vi "Test Set Base Path.vi"() -> ()   [LabVIEW 2021, in "Path Utilities.lvlib"]
doc: "Unit Test for \"Get In AppData Local.vi\"."
uses:
  Path Utilities.lvlib
panel:
  out "Pass":bool[](array[boolean])
  out "Result - System Paths with Base":path[](array[path])
  out "Expected - System Paths with Base":path[](array[path])
  in  "User Name":string="Thomas"
  out "error out":errorcluster
  in  "Base Path":path=path "Company/Application"
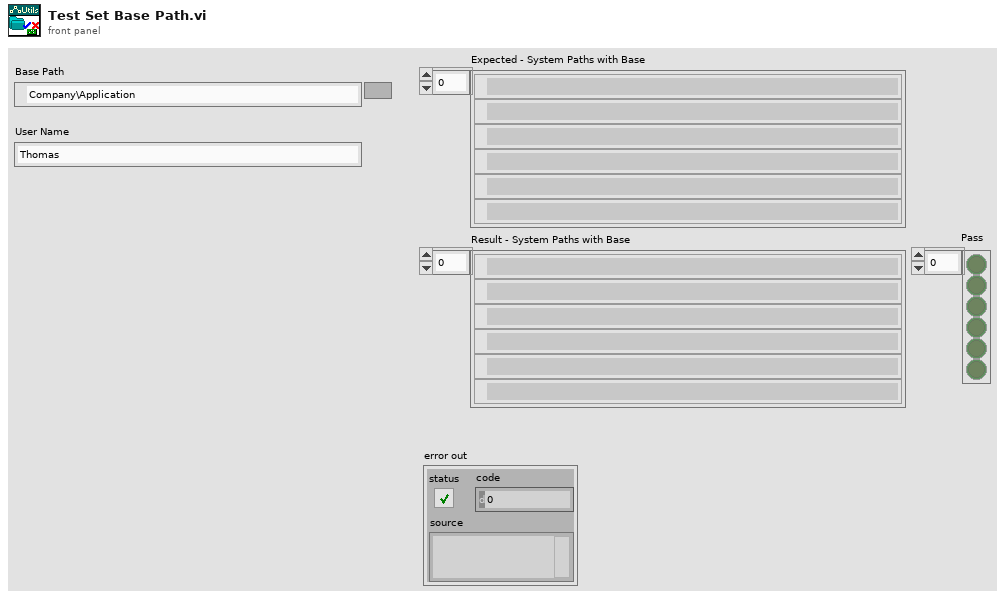
[diagram p1: front panel]
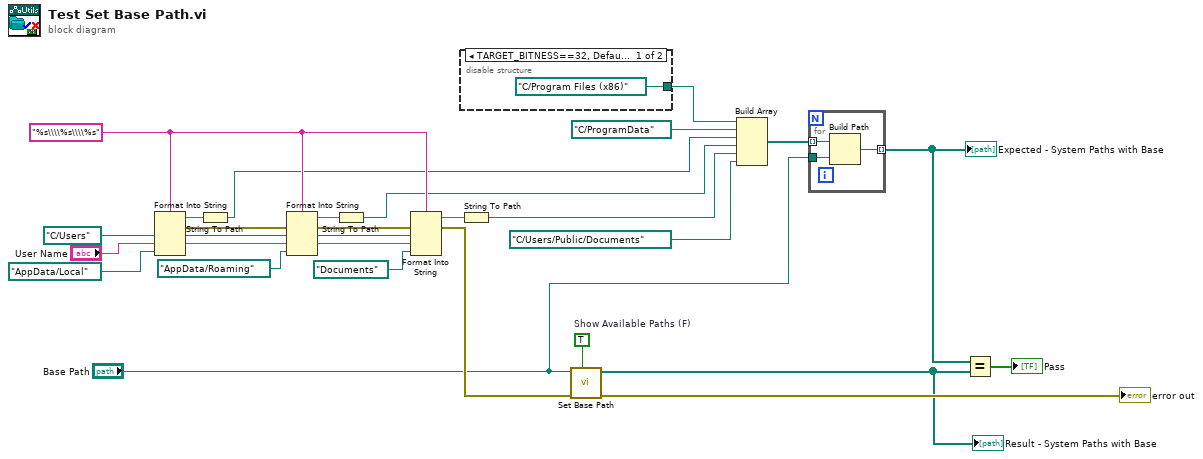
[diagram p0: block diagram]
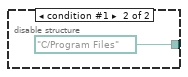
[diagram p2: hidden frame]
diagram:
  w1 = TRUE  # Show Available Paths (F)
  w16 = "%s\\\\%s\\\\%s" ("format string")
  w19 = path "C:/Users"
  n1 = Format Into String(format string=w16, w19, "User Name", path "AppData/Local") -> (resulting string=w24:string, error out=w23:errorcluster)  [unwired: 2 in]
  n2 = String To Path(string=w24) -> (path=w12:path)
  n3 = Format Into String(format string=w16, error in=w23, w19, "User Name", path "AppData/Roaming") -> (resulting string=w15:string, error out=w20:errorcluster)  [unwired: 1 in]
  n4 = String To Path(string=w15) -> (path=w11:path)
  n5 = Format Into String(format string=w16, error in=w20, w19, "User Name", path "Documents") -> (resulting string=w14:string, error out=w8:errorcluster)  [unwired: 1 in]
  n6 = disable-structure shown="TARGET_BITNESS==32, Default" {
    disable-tunnel: [path "C:/Program Files (x86)" path "C:/Program Files"] -> w21
    frame condition #0 (active) {
    }
    frame condition #1 {
    }
  }
  n7 = String To Path(string=w14) -> (path=w10:path)
  n8 = call "Set Base Path.vi"("Show Available Paths (F)"=w1, "error in (no error)"=w8, "Base Path"="Base Path") -> ("error out"=→"error out":errorcluster, "Available Paths"=w3:path[])  [unwired: 7 in]
  "Result - System Paths with Base" <- w3
  n9 = Build Array(w21, path "C:/ProgramData", w12, w11, w10, path "C:/Users/Public/Documents" ("base path")) -> (w7:path[])
  n10 = for {
    tunnel: w7 -> [w30] mode=indexing
    tunnel: "Base Path" -> [w29]
    tunnel: [w28] -> w4 mode=indexing
    n11 = Build Path(base path=w30, name or relative path=w29) -> (appended path=w28:path)
  }
  "Expected - System Paths with Base" <- w4
  n12 = Equal?(x=w4, y=w3) -> (x = y?=→"Pass":bool[])
